vi "Teleop.vi"(10 "Match Info":T1={"Autonomous Elapsed Seconds"=0.0, "TeleOp Elapsed Seconds"=0.0, "Disabled Elapsed Seconds"=0.0, "Visited Autonomous"=FALSE, "Visited TeleOp"=FALSE, "Visited Disabled"=FALSE, "Autonomous Settings"={"Autonomous Style"=enum."Independent", "VI Refnum"=refnum}}, 11 "Call Context":T2) -> ()   [LabVIEW 2012]
doc: "This VI is called for each TeleOp packet received from the DS where the robot is not disabled. It is often used to read from the joysticks and update I/O or to update setpoints for timed control loops. It should complete and return within 20 milliseconds or it may miss DS packets."
uses:
  <vilib>/Rock Robotics/WPI/DriverStation/WPI_DriverStationDerivedRobotMode.ctl
  <vilib>/Rock Robotics/WPI/DriverStation/WPI_DriverStationMatch Info.ctl
  Begin/Robot Global Data.vi
  Begin/Global Refnums.vi
  Begin/Global Variables.vi
  <vilib>/Rock Robotics/WPI/Joystick/WPI_JoystickGetSetRefNum.vi
panel:
  out "Numeric 1":dbl(slide) scale=0.0..100.0
  out "Boolean 2":bool
  out "Boolean 1":bool
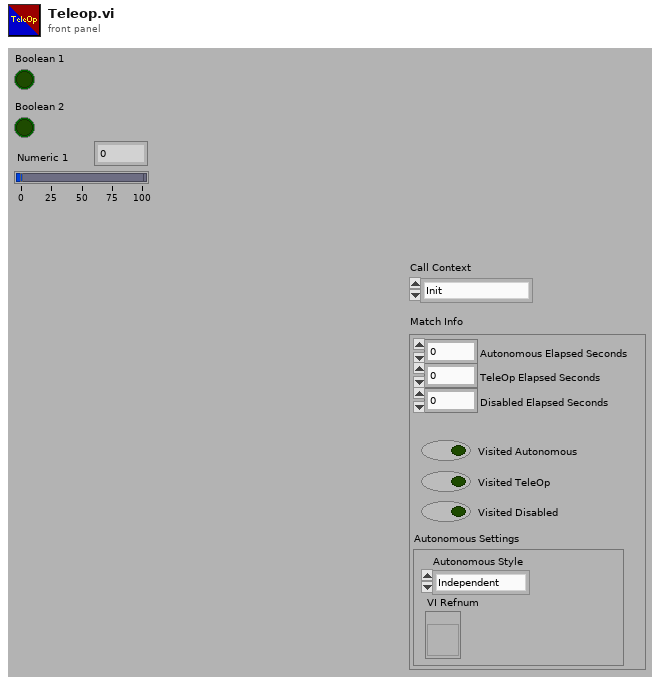
[diagram p1: front panel]
types:
  T1 = typedef "WPI_DriverStationMatch Info.ctl" = cluster{"Autonomous Elapsed Seconds":dbl, "TeleOp Elapsed Seconds":dbl, "Disabled Elapsed Seconds":dbl, "Visited Autonomous":bool, "Visited TeleOp":bool, "Visited Disabled":bool, "Autonomous Settings":cluster{"Autonomous Style":enum16{"Iterative", "Independent"}, "VI Refnum":refnum<vi>}}
  T2 = typedef "WPI_DriverStationDerivedRobotMode.ctl" = enum16{"Init", "Execute", "Stop"}
  T3 = typedef "WPI_JoystickDevRef.ctl" = cluster{"Device":T4}
  T4 = typedef "WPI_JoystickDeviceEnum.ctl" = enum16{"USB 1", "USB 2", "USB 3", "USB 4", "Kinect 1", "Kinect 2"}
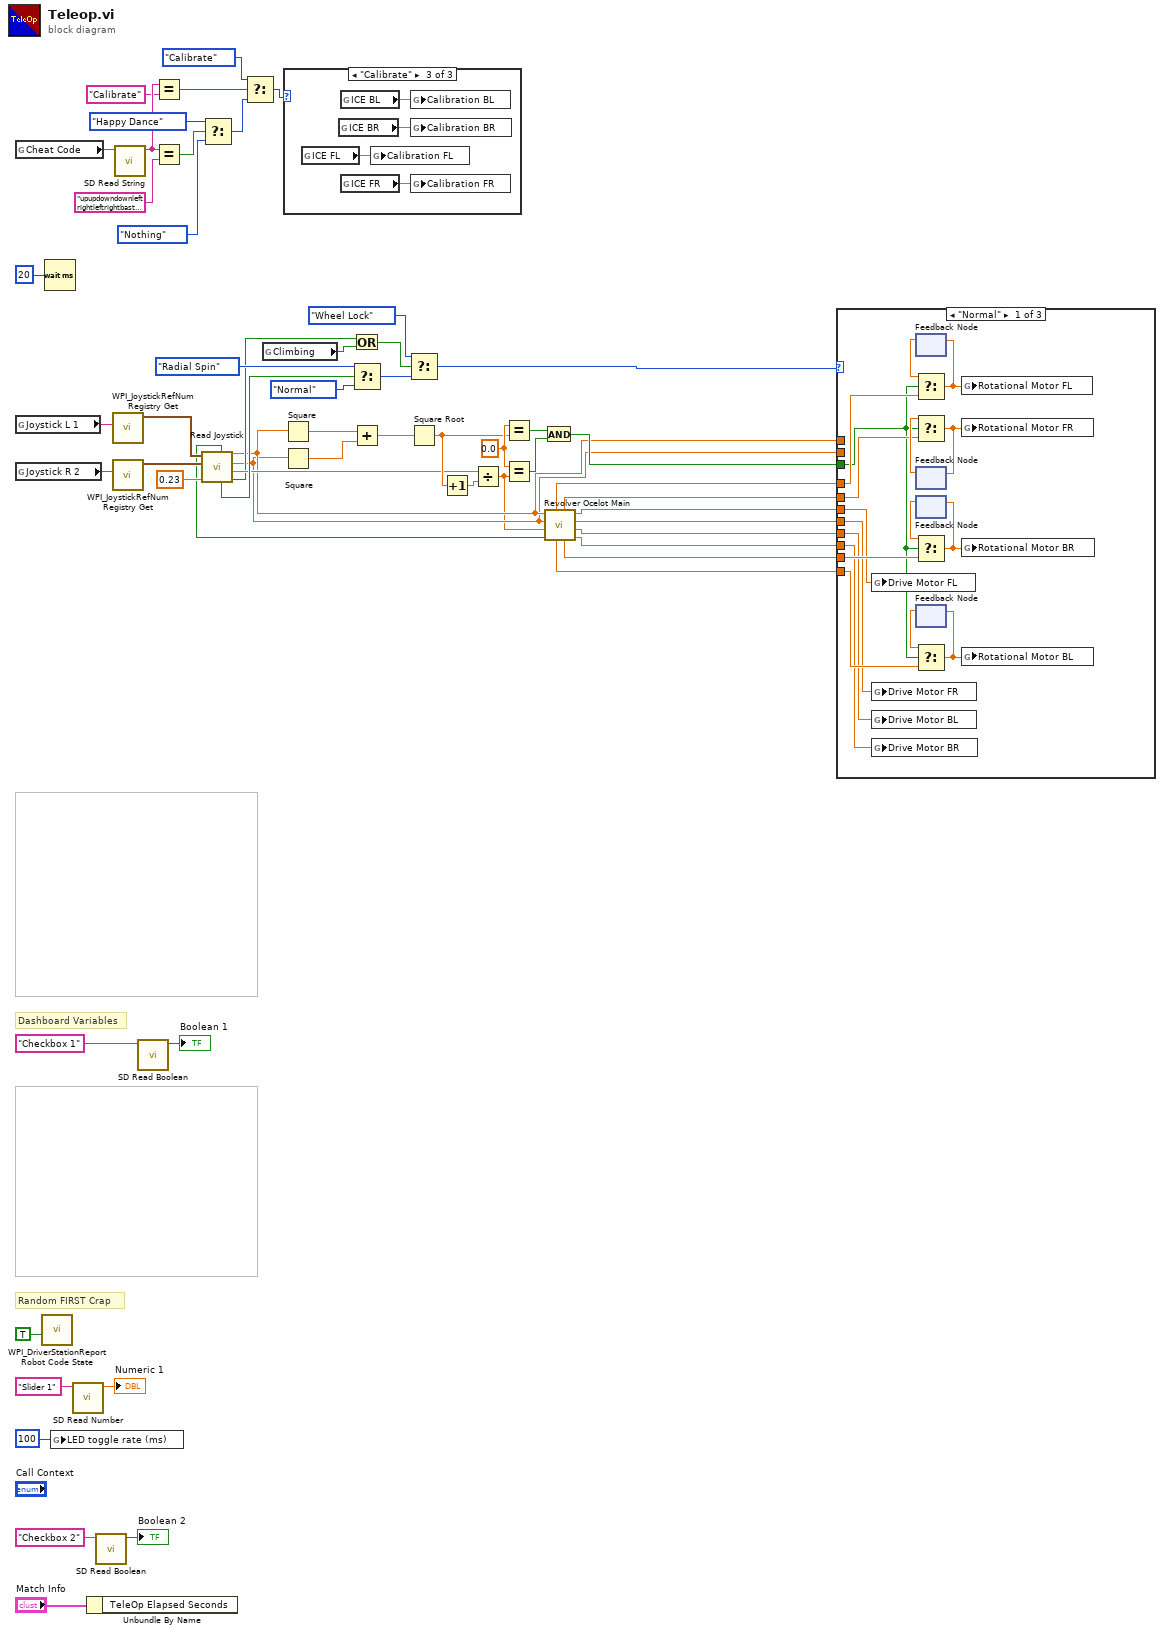
[diagram p0: block diagram]
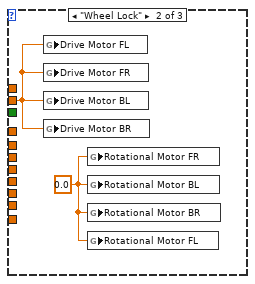
[diagram p2: hidden frame]
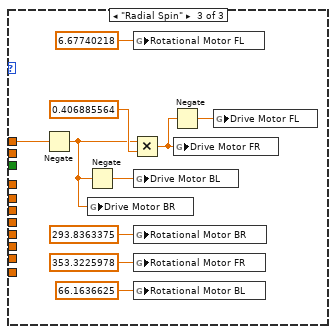
[diagram p3: hidden frame]
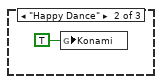
[diagram p5: hidden frame]
diagram:
  w34 = 0.0 ("x")
  # "Dashboard Variables"
  # "Random FIRST Crap"
  n1 = global read "Global Refnums.vi" "Cheat Code"() -> (w47:string)
  n2 = global read "Global Refnums.vi" "Joystick L 1"() -> (w43:string)
  n3 = global read "Global Refnums.vi" "Joystick R 2"() -> (w42:string)
  n4 = call <vilib>:"WPI_DriverStationReport Robot Code State.vi"("TeleOp"=TRUE ("Autonomous")) -> ()  [unwired: 10 in, 1 out]
  n5 = Wait (ms)(milliseconds to wait=u32 20) -> ()  [unwired: 1 out]
  n6 = global write "Robot Global Data.vi" "LED toggle rate (ms)"(u32 100 ("LED ms toggle rate")) -> ()
  n7 = call <vilib>:"SD Read Number.vi"("Name"="Slider 1" ("refnum name")) -> ("Numeric"=→"Numeric 1":dbl)  [unwired: 8 in, 2 out]
  n8 = Unbundle By Name("Match Info") -> ()  [unwired: 1 out]
  n9 = call <vilib>:"SD Read Boolean.vi"("Name"="Checkbox 2" ("refnum name")) -> ("Boolean"=→"Boolean 2":bool)  [unwired: 8 in, 2 out]
  n10 = call <vilib>:"WPI_JoystickRefNum Registry Get.vi"("refnum name"=w43) -> ("JoystickDevRef"=w44:T3)  [unwired: 9 in, 1 out]
  n11 = call <vilib>:"WPI_JoystickRefNum Registry Get.vi"("refnum name"=w42) -> ("JoystickDevRef"=w45:T3)  [unwired: 9 in, 1 out]
  n12 = call <vilib>:"SD Read String.vi"("Name"=w47) -> ("String"=w48:string)  [unwired: 8 in, 2 out]
  n13 = call <vilib>:"SD Read Boolean.vi"("Name"="Checkbox 1" ("refnum name")) -> ("Boolean"=→"Boolean 1":bool)  [unwired: 8 in, 2 out]
  n14 = Equal?(x=w48, y="Calibrate") -> (x = y?=w30:bool)
  n15 = Equal?(x=w48, y="upupdowndownleftrightleftrightbastart") -> (x = y?=w26:bool)
  n16 = call "Read Joystick.vi"("Joystick Deadbanded Value (default of 0.1)"=0.23, "Joystick R 2 DevRef"=w45, "Joystick L 1 DevRef"=w44) -> ("Wheel Lock"=w16:bool, "Joystick R 2 X Axis"=w17:dbl, "Joystick L 1 Y Axis"=w11:dbl, "Joystick L 1 X Axis"=w12:dbl, "Radial Spin"=w21:bool, "Revolver"=w1:bool)  [unwired: 3 in]
  n17 = Select(t=enum16{"Nothing", "Happy Dance", "Calibrate"}."Happy Dance", s=w26, f=enum16{"Nothing", "Happy Dance", "Calibrate"}."Nothing") -> (s? t:f=w24:enum16{"Nothing", "Happy Dance", "Calibrate"})
  n18 = Select(t=enum16{"Nothing", "Happy Dance", "Calibrate"}."Calibrate", s=w30, f=w24) -> (s? t:f=w28:enum16{"Nothing", "Happy Dance", "Calibrate"})
  n19 = global read "Global Variables.vi" "Climbing"() -> (w14:bool)
  n20 = Square(x=w12) -> (x^2=w39:dbl)
  n21 = Square(x=w11) -> (x^2=w40:dbl)
  n22 = case shown="\"Calibrate\"" w28 {
    frame "Nothing", Default {
    }
    frame "Happy Dance" {
      n23 = global write "Global Variables.vi" "Konami"(TRUE) -> ()
    }
    frame "Calibrate" {
      n24 = global read "Global Variables.vi" "ICE FL"() -> (w60:dbl)
      n25 = global read "Global Variables.vi" "ICE BR"() -> (w61:dbl)
      n26 = global read "Global Variables.vi" "ICE BL"() -> (w62:dbl)
      n27 = global read "Global Variables.vi" "ICE FR"() -> (w59:dbl)
      n28 = global write "Global Variables.vi" "Calibration FL"(w60) -> ()
      n29 = global write "Global Variables.vi" "Calibration BL"(w62) -> ()
      n30 = global write "Global Variables.vi" "Calibration BR"(w61) -> ()
      n31 = global write "Global Variables.vi" "Calibration FR"(w59) -> ()
    }
  }
  n32 = Or(x=w16, y=w14) -> (x .or. y?=w15:bool)
  n33 = Select(t=enum16{"Normal", "Wheel Lock", "Radial Spin"}."Radial Spin", s=w21, f=enum16{"Normal", "Wheel Lock", "Radial Spin"}."Normal") -> (s? t:f=w22:enum16{"Normal", "Wheel Lock", "Radial Spin"})
  n34 = Add(x=w39, y=w40) -> (x+y=w38:dbl)
  n35 = Select(t=enum16{"Normal", "Wheel Lock", "Radial Spin"}."Wheel Lock", s=w15, f=w22) -> (s? t:f=w13:enum16{"Normal", "Wheel Lock", "Radial Spin"})
  n36 = Square Root(x=w38) -> (sqrt(x)=w32:dbl)
  n37 = Increment(x=w32) -> (x+1=w33:dbl)
  n38 = Divide(x=w17, y=w33) -> (x/y=w10:dbl)
  n39 = Equal?(x=w34, y=w32) -> (x = y?=w36:bool)
  n40 = Equal?(x=w34, y=w10) -> (x = y?=w35:bool)
  n41 = And(x=w36, y=w35) -> (x .and. y?=w37:bool)
  n42 = call "Revolver Ocelot Main.vi"("Ocelot"=w1, "Z"=w10, "Y"=w11, "X"=w12) -> ("BRD"=w2:dbl, "BLD"=w3:dbl, "FRD"=w4:dbl, "FLD"=w5:dbl, "BRS"=w6:dbl, "FRS"=w8:dbl, "BLS"=w7:dbl, "FLS"=w9:dbl)
  n43 = case shown="\"Normal\"" w13 {
    tunnel: w6 -> [w75 _ _]
    tunnel: w7 -> [w74 _ _]
    tunnel: w8 -> [w73 _ _]
    tunnel: w9 -> [w70 _ _]
    tunnel: w37 -> [w67 _ _]
    tunnel: w5 -> [w66 _ _]
    tunnel: w4 -> [w65 _ _]
    tunnel: w3 -> [w64 _ _]
    tunnel: w2 -> [w63 _ _]
    tunnel: w12 -> [_ _ w86]
    tunnel: w11 -> [_ w80 _]
    frame "Normal" {
      n44 = global write "Global Variables.vi" "Drive Motor FL"(w66) -> ()
      n45 = global write "Global Variables.vi" "Drive Motor FR"(w65) -> ()
      n46 = global write "Global Variables.vi" "Drive Motor BL"(w64) -> ()
      n47 = global write "Global Variables.vi" "Drive Motor BR"(w63) -> ()
      n48 = feedback #1() -> (w79:dbl)  [unwired: 1 in]
      n49 = Select(t=w79, s=w67, f=w70) -> (s? t:f=w69:dbl)
      n50 = feedback-in #1(w69) -> ()
      n51 = feedback #2() -> (w78:dbl)  [unwired: 1 in]
      n52 = Select(t=w78, s=w67, f=w73) -> (s? t:f=w72:dbl)
      n53 = feedback-in #2(w72) -> ()
      n54 = feedback #3() -> (w76:dbl)  [unwired: 1 in]
      n55 = Select(t=w76, s=w67, f=w75) -> (s? t:f=w68:dbl)
      n56 = feedback-in #3(w68) -> ()
      n57 = feedback #4() -> (w77:dbl)  [unwired: 1 in]
      n58 = Select(t=w77, s=w67, f=w74) -> (s? t:f=w71:dbl)
      n59 = feedback-in #4(w71) -> ()
      n60 = global write "Global Variables.vi" "Rotational Motor FL"(w69) -> ()
      n61 = global write "Global Variables.vi" "Rotational Motor FR"(w72) -> ()
      n62 = global write "Global Variables.vi" "Rotational Motor BR"(w68) -> ()
      n63 = global write "Global Variables.vi" "Rotational Motor BL"(w71) -> ()
    }
    frame "Wheel Lock" {
      w81 = 0.0
      n64 = global write "Global Variables.vi" "Drive Motor FL"(w80) -> ()
      n65 = global write "Global Variables.vi" "Drive Motor FR"(w80) -> ()
      n66 = global write "Global Variables.vi" "Drive Motor BL"(w80) -> ()
      n67 = global write "Global Variables.vi" "Drive Motor BR"(w80) -> ()
      n68 = global write "Global Variables.vi" "Rotational Motor FR"(w81) -> ()
      n69 = global write "Global Variables.vi" "Rotational Motor BL"(w81) -> ()
      n70 = global write "Global Variables.vi" "Rotational Motor BR"(w81) -> ()
      n71 = global write "Global Variables.vi" "Rotational Motor FL"(w81) -> ()
    }
    frame "Radial Spin" {
      n72 = Negate(x=w86) -> (-x=w82:dbl)
      n73 = Negate(x=w82) -> (-x=w83:dbl)
      n74 = global write "Global Variables.vi" "Drive Motor BR"(w82) -> ()
      n75 = Multiply(x=w82, y=0.406885564) -> (x*y=w85:dbl)
      n76 = global write "Global Variables.vi" "Rotational Motor FL"(6.67740218) -> ()
      n77 = global write "Global Variables.vi" "Drive Motor BL"(w83) -> ()
      n78 = global write "Global Variables.vi" "Rotational Motor BR"(293.8363375) -> ()
      n79 = global write "Global Variables.vi" "Rotational Motor FR"(353.3225978) -> ()
      n80 = global write "Global Variables.vi" "Rotational Motor BL"(66.1636625) -> ()
      n81 = Negate(x=w85) -> (-x=w84:dbl)
      n82 = global write "Global Variables.vi" "Drive Motor FR"(w85) -> ()
      n83 = global write "Global Variables.vi" "Drive Motor FL"(w84) -> ()
    }
  }
